vi "UIRef.vi"(8 "error in":errorcluster, 11 "node in":refnum<class "Page.lvclass">) -> (0 "error out":errorcluster, 2 "VI refnum":refnum<vi>, 3 "node out":refnum<class "Page.lvclass">)   [LabVIEW 2015, in "Page.lvclass"]
doc: "Stores the static reference to the UI of the node."
uses:
  Page.lvclass
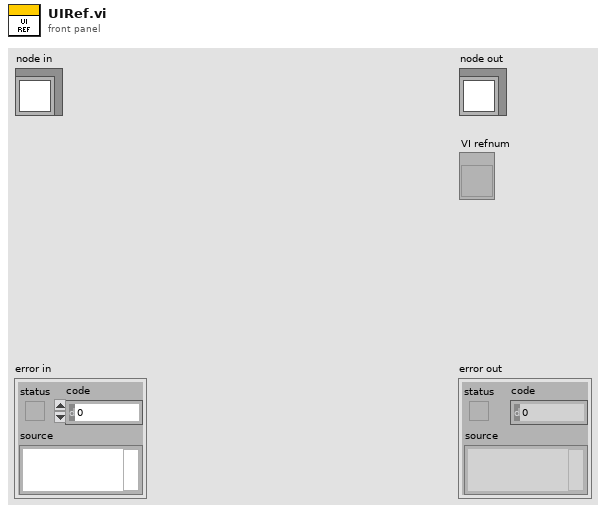
[diagram p1: front panel]
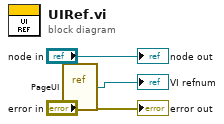
[diagram p0: block diagram]
diagram:
  n1 = vi-ref "PageUI.vi"() -> (→"VI refnum":refnum<vi>)
  "error out" <- "error in"
  "node out" <- "node in"
